vi "Power Law Model VI.vi"(3 "output control":T1, 4 "data":variant, 5 "X":dbl[](array[numeric]), 6 "a":dbl[](array[numeric])) -> (0 "error out":errorcluster, 1 "f'(X,a)":dbl[][](array[numeric]), 2 "f(X,a)":dbl[](array[numeric]))   [LabVIEW 2022 SP3]
doc: "Implements an ellipse model function to be passed to the Nonlinear Curve Fit.vi."
uses:
  <vilib>/gmath/NumericalOptimization/LM_output select.ctl
  <vilib>/gmath/NI_Gmath.lvlib
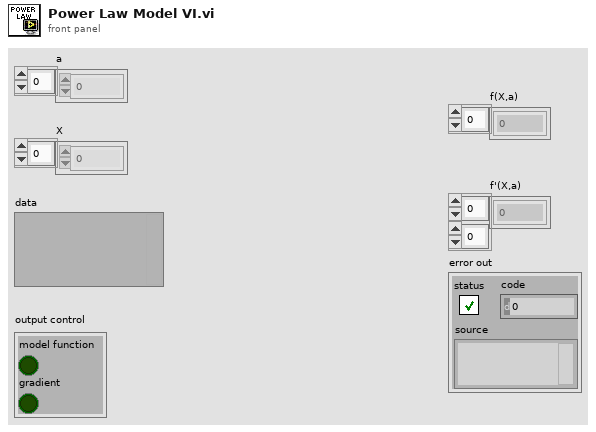
[diagram p1: front panel]
types:
  T1 = typedef "NI_Gmath.lvlib/LM_output select.ctl" = cluster{"model function":bool, "gradient":bool}
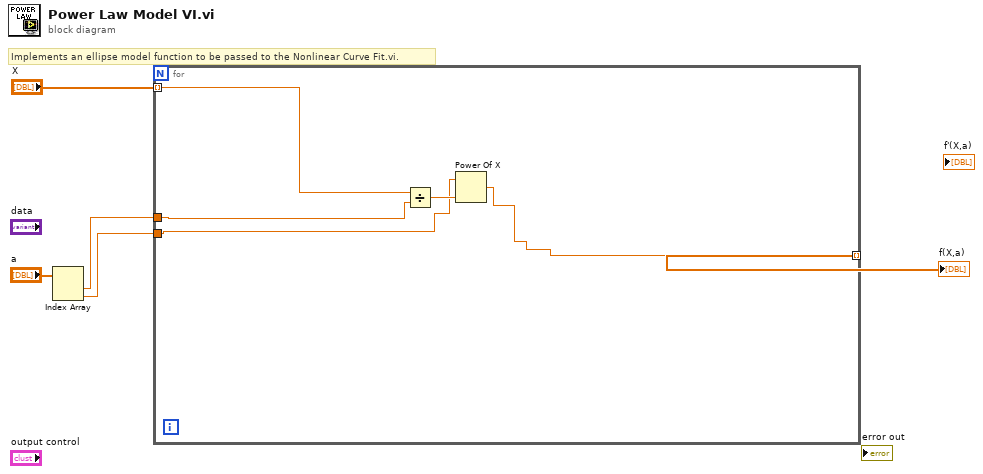
[diagram p0: block diagram]
diagram:
  # "Implements an ellipse model function to be passed to the Nonlinear Curve Fit.vi."
  n1 = Index Array(array="a") -> (element #1=w2:dbl, element #2=w1:dbl)  [unwired: 2 in]
  n2 = for {
    tunnel: [w6] -> w5 mode=indexing
    tunnel: "X" -> [w9] mode=indexing
    tunnel: w2 -> [w10]
    tunnel: w1 -> [w7]
    n3 = Divide(x=w9, y=w10) -> (x/y=w8:dbl)
    n4 = Power Of X(1:w8, 2:w7) -> (0:w6:dbl)
  }
  "f(X,a)" <- w5
